vi "Host_SuspensionCurrentCheck.vi"() -> ()   [LabVIEW 2014]
uses:
  <vilib>/FPGAPlugInAG/PCIe-7851R/niLvFpga_Open_PCIe-7851R.vi
  <vilib>/rvi/interface/common/dynamic/niFpgaDynamicAddResources.vi
  <vilib>/Utility/error.llb/Error Cluster From Error Code.vi
  <vilib>/rvi/errors/niLvFpgaAdjustHostInterfaceError.vi
  <vilib>/rvi/interface/nirviOpenFPGA/nirviOpenFPGA.xnode
  FPGA Bitfiles/XZFPGAWithinHopp_FPGATarget_FPGASuspensionCu_ZLyBgXDLLGY.lvbitx
  <vilib>/rvi/interface/nirviReadWriteControl/nirviReadWriteControl.xnode
  <vilib>/rvi/interface/nirviMethod/nirviMethod.xnode
  <vilib>/rvi/interface/Simulation/niFpgaSimulationCallBeginRW.vi
  <vilib>/FPGAPlugInAG/Dynamic/niLvFpga_ReadFifo_Dynamic.vi
  <vilib>/rvi/errors/niLvFpgaMergeErrorWithErrorCode.vi
  NiFpgaLv.dll
panel:
  in  "StepPulseIndex":u32
  in  "SampleSleep us":i32
  in  "StepIn?":bool
  in  "StepInNum":i32
  in  "SampleNumPerStepIn":i32
  in  "SampleNumAfter":i32
  out "elapsed_sec":dbl
  out "PtsGetNum":u32
  out "Finished?":bool
  out "Current":i16[](graph)
  out "ZPos":i16(graph)
  in  "stop":bool
  in  "threshold":sgl
  in  "sleep us":u32
  in  "Offset":i16
  in  "SampleNum":i32
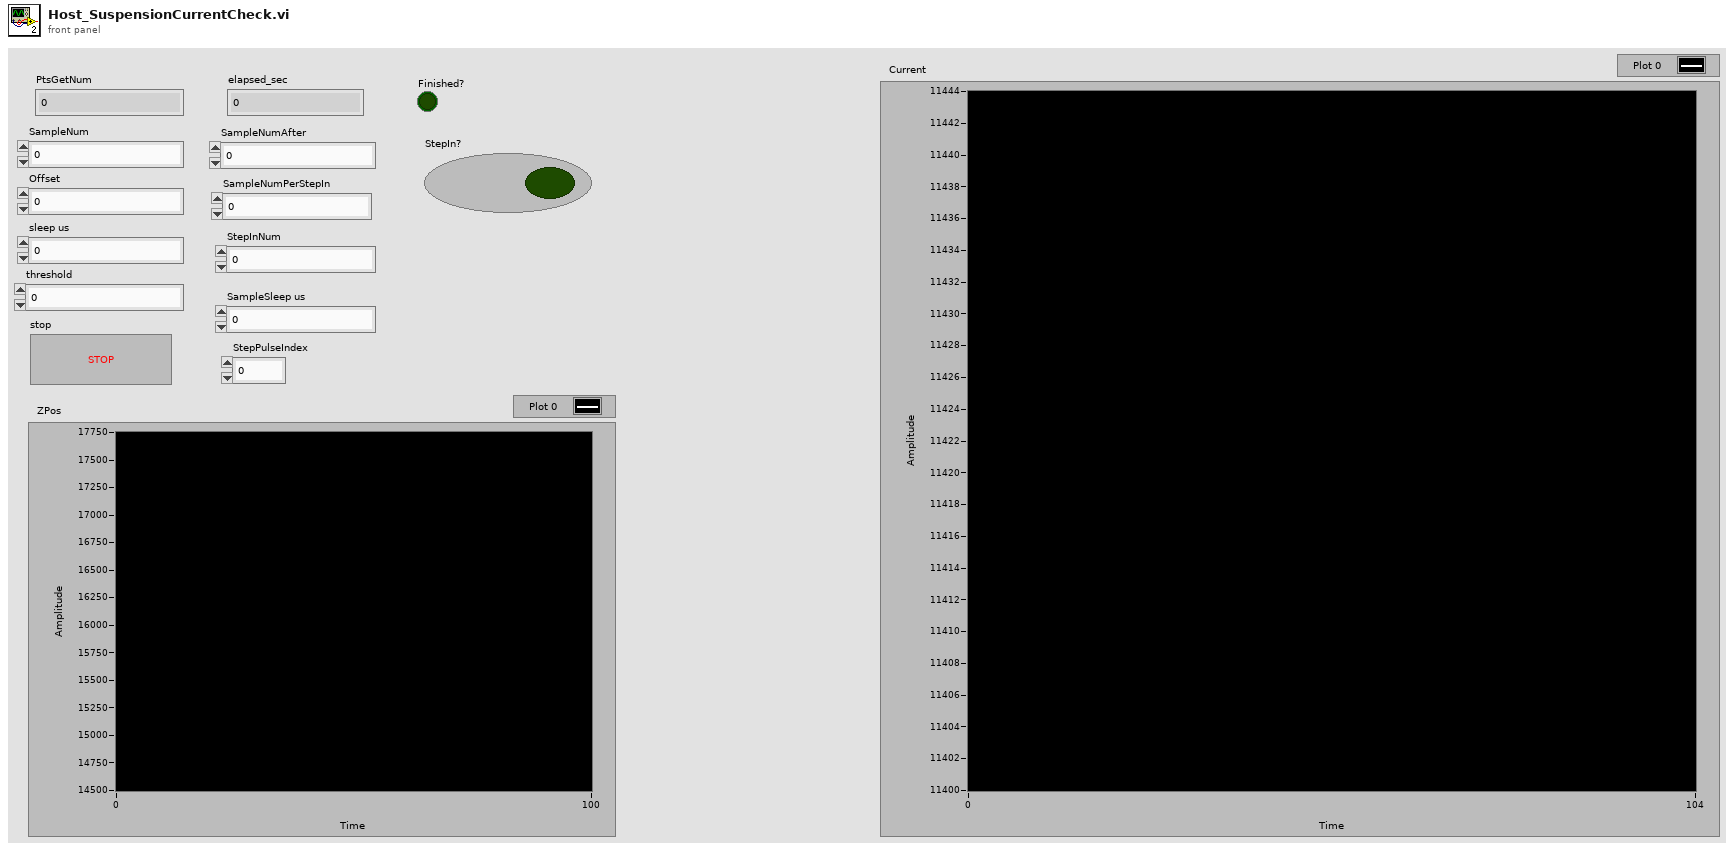
[diagram p1: front panel]
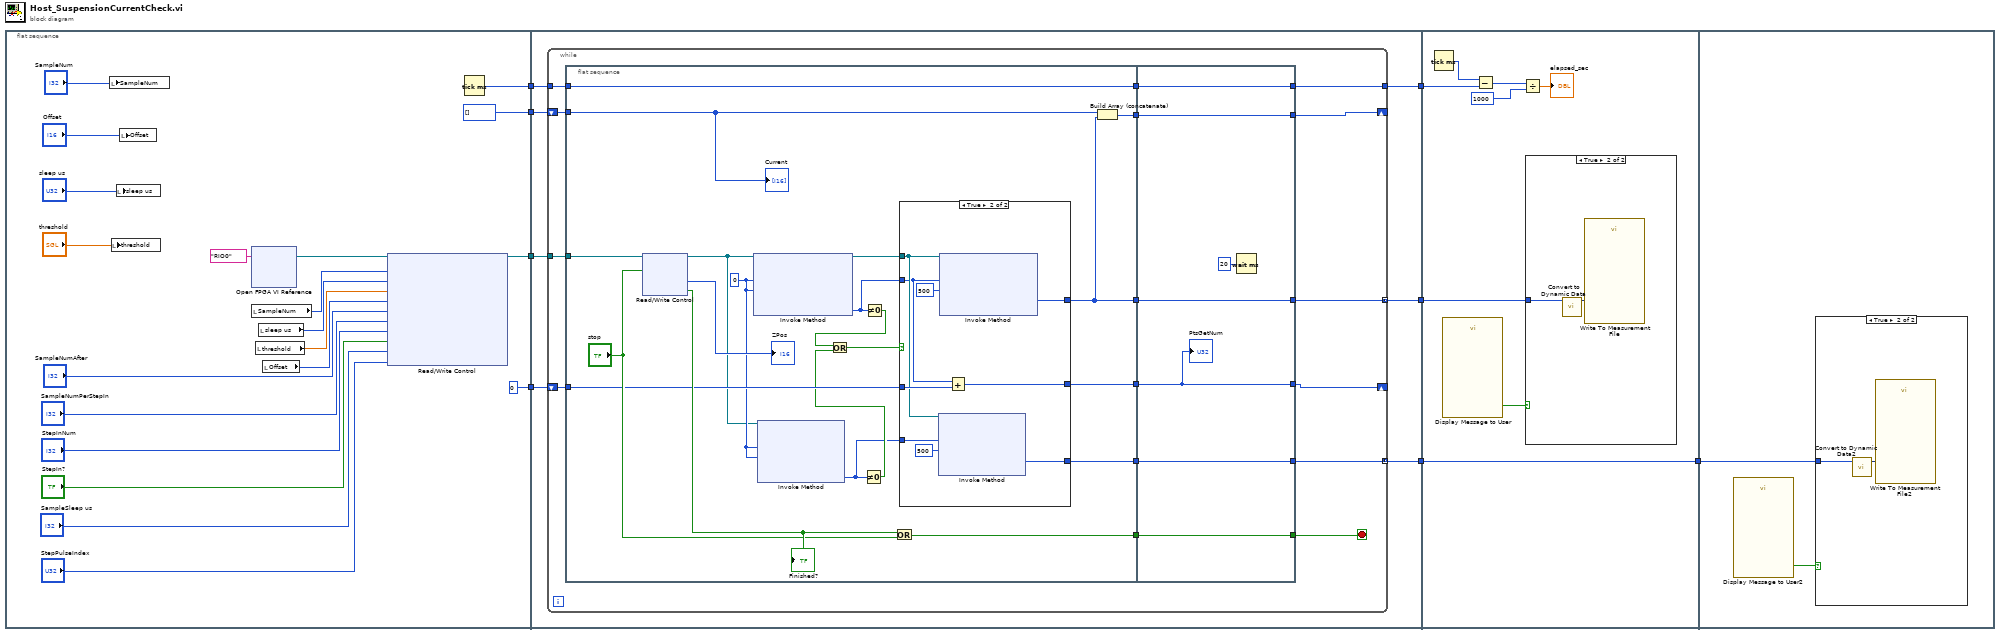
[diagram p0: block diagram]
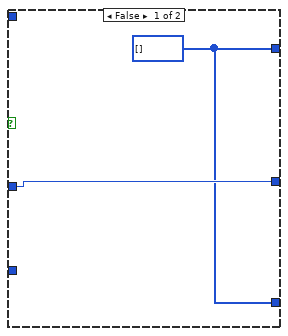
[diagram p2: hidden frame]
diagram:
  n1 = flat-sequence {
    tunnel: [w22] -> w8
    tunnel: [i16[] []] -> w7
    tunnel: [0] -> w5
    tunnel: [w15] -> w4
    tunnel: w8 -> [w35]
    tunnel: w7 -> [w34]
    tunnel: [w33] -> w6
    tunnel: w5 -> [w32]
    tunnel: w4 -> [w31]
    tunnel: [w30] -> w3
    tunnel: [w29] -> w2
    tunnel: w6 -> [w96]
    tunnel: w3 -> [w94]
    tunnel: w2 -> [w90]
    tunnel: [w90] -> w1
    tunnel: w1 -> [w100]
    frame #0 {
      n2 = local write "SampleNum"("SampleNum") -> ()
      n3 = local write "threshold"("threshold") -> ()
      n4 = local write "sleep us"("sleep us") -> ()
      n5 = local write "Offset"("Offset") -> ()
      n6 = xnode ("Open FPGA VI Reference")("resource name"=tag "RIO0") -> ("FPGA VI Reference Out"=w23:refnum<k20>)  [unwired: 1 in, 1 out]
      n7 = local read "SampleNum"() -> (w21:i32)
      n8 = local read "threshold"() -> (w19:sgl)
      n9 = local read "sleep us"() -> (w20:u32)
      n10 = local read "Offset"() -> (w18:i16)
      n11 = xnode "Read/Write Control"("FPGA VI Reference In"=w23, "SampleNumAfterApproached"=w21, "sleep us"=w20, "threshold"=w19, "Offset"=w18, "SampleNumAfterBack"="SampleNumAfter", "SampleNumPerStepIn"="SampleNumPerStepIn", "StepInNum"="StepInNum", "StepIn?"="StepIn?", "SampleSleep us"="SampleSleep us", "StepPulseIndex"="StepPulseIndex") -> ("FPGA VI Reference Out"=w22:refnum<k20>)  [unwired: 1 in, 1 out]
      n12 = Tick Count (ms)() -> (millisecond timer value=w15:u32)
    }
    frame #1 {
      n13 = while {
        tunnel: w35 -> [w51]
        shift-right: [w46] -> _
        shift-left: w34 -> [w50]
        tunnel: [w48] -> w33 mode=concatenating
        shift-right: [w41] -> _
        shift-left: w32 -> [w43]
        tunnel: w31 -> [w40]
        tunnel: [w38] -> w30
        tunnel: [w36] -> w29 mode=concatenating
        stop <- w44 stop-if-true
        n14 = flat-sequence {
          tunnel: w51 -> [w71]
          tunnel: w50 -> [w66]
          tunnel: [w68] -> w49
          tunnel: [w67] -> w47
          tunnel: [w62] -> w45
          tunnel: w43 -> [w61]
          tunnel: [w60] -> w42
          tunnel: w40 -> [w59]
          tunnel: [w59] -> w39
          tunnel: [w58] -> w37
          tunnel: [w89] -> w48
          tunnel: w49 -> [w89]
          tunnel: [w88] -> w46
          tunnel: w47 -> [w88]
          tunnel: [w87] -> w44
          tunnel: w45 -> [w87]
          tunnel: [w85] -> w41
          tunnel: w42 -> [w85]
          tunnel: w39 -> [w84]
          tunnel: [w84] -> w38
          tunnel: w37 -> [w83]
          tunnel: [w83] -> w36
          frame #0 {
            w57 = u32 0 ("Number of Elements")
            n15 = xnode "Read/Write Control"("FPGA VI Reference In"=w71, "stop"="stop") -> ("FPGA VI Reference Out"=w53:refnum<k20>, "ZPos"=→"ZPos":i16, "Finished?"=w64:bool)  [unwired: 1 in, 1 out]
            "Finished?" <- w64
            n16 = xnode "Invoke Method"("FPGA VI Reference In"=w53, "Number of Elements"=w57, "Timeout (ms)"=w57) -> ("FPGA VI Reference Out"=w70:refnum<k20>, "Elements Remaining"=w69:u32)  [unwired: 1 in, 2 out]
            n17 = xnode "Invoke Method"("FPGA VI Reference In"=w53, "Number of Elements"=w57, "Timeout (ms)"=w57) -> ("Elements Remaining"=w52:u32)  [unwired: 1 in, 3 out]
            n18 = Not Equal To 0?(x=w52) -> (x != 0?=w55:bool)
            n19 = Not Equal To 0?(x=w69) -> (x != 0?=w56:bool)
            n20 = Or(x=w56, y=w55) -> (x .or. y?=w54:bool)
            n21 = Or(x=w64, y="stop") -> (x .or. y?=w62:bool)
            n22 = case shown="True" w54 {
              tunnel: w70 -> [_ w78]
              tunnel: w69 -> [_ w77]
              tunnel: [w72 w81] -> w68
              tunnel: w61 -> [w73 w80]
              tunnel: [w73 w79] -> w60
              tunnel: [w72 w75] -> w58
              tunnel: w52 -> [_ w74]
              frame False {
                w72 = i16[] [] ("Data")
              }
              frame True {
                n23 = xnode "Invoke Method"("FPGA VI Reference In"=w78, "Number of Elements"=w74, "Timeout (ms)"=500) -> ("Data"=w75:i16[])  [unwired: 1 in, 3 out]
                n24 = xnode "Invoke Method"("FPGA VI Reference In"=w78, "Number of Elements"=w77, "Timeout (ms)"=500) -> ("Data"=w81:i16[])  [unwired: 1 in, 3 out]
                n25 = Add(x=w77, y=w80) -> (x+y=w79:u32)
              }
            }
            n26 = Build Array (concatenate)(w66, w68) -> (w67:i16[])
            "Current" <- w66
          }
          frame #1 {
            n27 = Wait (ms)(milliseconds to wait=u32 20) -> ()  [unwired: 1 out]
            "PtsGetNum" <- w85
          }
        }
      }
    }
    frame #2 {
      n28 = Tick Count (ms)() -> (millisecond timer value=w95:u32)
      n29 = call "Display Message to User"() -> ("OK"=w97:bool)  [unwired: 10 in, 1 out]
      n30 = Subtract(x=w95, y=w94) -> (x-y=w93:u32)
      n31 = Divide(x=w93, y=u32 1000) -> (x/y=→"elapsed_sec":dbl)
      n32 = case shown="True" w97 {
        tunnel: w96 -> [_ w99]
        frame False {
        }
        frame True {
          n33 = call "Convert to Dynamic Data"("Array"=w99) -> ("Dynamic Data Type"=w98:dynamicdata)  [unwired: 3 in]
          n34 = call "Write To Measurement File"("Signals"=w98) -> ()  [unwired: 16 in, 3 out]
        }
      }
    }
    frame #3 {
      n35 = call "Display Message to User2"() -> ("OK"=w101:bool)  [unwired: 10 in, 1 out]
      n36 = case shown="True" w101 {
        tunnel: w100 -> [_ w103]
        frame False {
        }
        frame True {
          n37 = call "Convert to Dynamic Data2"("Array"=w103) -> ("Dynamic Data Type"=w102:dynamicdata)  [unwired: 3 in]
          n38 = call "Write To Measurement File2"("Signals"=w102) -> ()  [unwired: 16 in, 3 out]
        }
      }
    }
  }
